vi "Zones Distance Under Value.vi"(9 "Value":i32=10000, 10 "Range":i32[](array[numeric]), 11 "Manhattan Distances":i32[][][](array[numeric])) -> (3 "Numeric":i32)   [LabVIEW 2019]
doc: "Given manhattan distances generated from a list of points, and a range of values to calculate distances from. This VI doesn't care what the values of the range are, just that it's the same length as the point matrices used to generate the Manhattan Distance array.\n\nThis VI will return the number of spaces whose total manhattan distance (i.e. distance to all points given from the coordinates) is under the provided value."
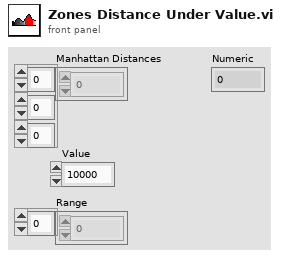
[diagram p1: front panel]
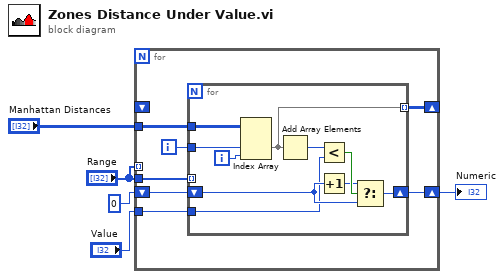
[diagram p0: block diagram]
diagram:
  n1 = for {
    tunnel: "Manhattan Distances" -> [w12]
    tunnel: "Range" -> [_] mode=indexing
    tunnel: "Range" -> [w11]
    shift-right: [w9] -> w4
    shift-left: 0 -> [w10]
    shift-right: [w8] -> _
    shift-left: _ -> [_]
    tunnel: "Value" -> [w6]
    i -> [w7]
    n2 = for {
      tunnel: w12 -> [w22]
      tunnel: w11 -> [_] mode=indexing
      shift-right: [w17] -> w9
      shift-left: w10 -> [w18]
      tunnel: [w16] -> w8 mode=indexing
      tunnel: w7 -> [w15]
      tunnel: w6 -> [w13]
      i -> [w14]
      n3 = Index Array(array=w22, index (dim 1)=w15, index (dim 2)=w14) -> (element=w16:i32[])  [unwired: 1 in]
      n4 = Add Array Elements(numeric array=w16) -> (sum=w21:i32)
      n5 = Less?(x=w21, y=w13) -> (x < y?=w20:bool)
      n6 = Increment(x=w18) -> (x+1=w19:i32)
      n7 = Select(t=w19, s=w20, f=w18) -> (s? t:f=w17:i32)
    }
  }
  "Numeric" <- w4
